vi "Practica 3.vi"() -> ()   [LabVIEW 2019]
panel:
  out "Temperatura leída":dbl
  in  "Temperatura mínima":dbl=30.0 format="%#_13g"
  in  "Temperatura máxima":dbl=36.0 format="%#_13g"
  in  "?":bool
  # "Práctica #3. Construcción de instrumentos virtuales \npara el control de variables físicas"
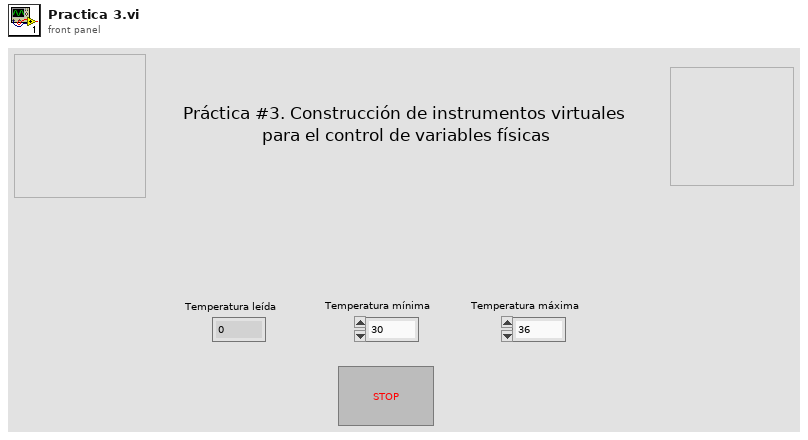
[diagram p1: front panel]
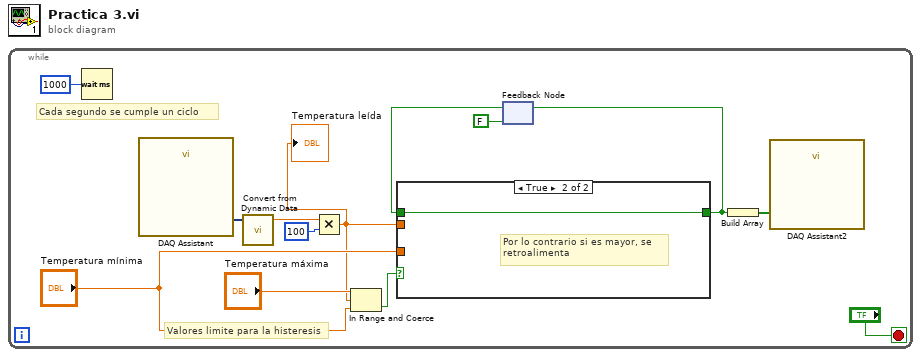
[diagram p0: block diagram]
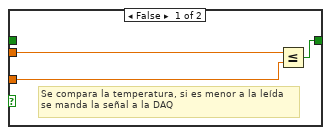
[diagram p2: hidden frame]
diagram:
  n1 = while {
    stop <- "?" stop-if-true
    # "Cada segundo se cumple un ciclo"
    # "Valores limite para la histeresis"
    n2 = Wait (ms)(milliseconds to wait=u32 1000) -> ()  [unwired: 1 out]
    n3 = call "DAQ Assistant"() -> ("data"=w7:dynamicdata)  [unwired: 17 in, 2 out]
    n4 = call "Convert from Dynamic Data"("Dynamic Data Type"=w7) -> ("Scalar"=w2:dbl)  [unwired: 3 in]
    n5 = Multiply(x=w2, y=100) -> (x*y=w1:dbl)
    "Temperatura leída" <- w1
    n6 = In Range and Coerce(upper limit="Temperatura máxima", x=w1, lower limit="Temperatura mínima") -> (In Range?=w12:bool)  [unwired: 1 out]
    n7 = feedback #1(FALSE) -> (w9:bool)
    n8 = case shown="True" w12 {
      tunnel: w1 -> [w16 _]
      tunnel: "Temperatura mínima" -> [w15 _]
      tunnel: [w14 w17] -> w6
      tunnel: w9 -> [_ w17]
      frame False {
        # "Se compara la temperatura, si es menor a la leída\nse manda la señal a la DAQ"
        n9 = Less Or Equal?(x=w16, y=w15) -> (x <= y?=w14:bool)
      }
      frame True {
        # "Por lo contrario si es mayor, se \nretroalimenta"
      }
    }
    n10 = feedback-in #1(w6) -> ()
    n11 = Build Array(w6) -> (w5:bool[])
    n12 = call "DAQ Assistant2"("data"=w5) -> ()  [unwired: 17 in, 2 out]
  }
